vi "TestSimpleVISAconnection.vi"() -> ()   [LabVIEW 2015]
panel:
  out "read buffer":string
  in  "wr":bool
  in  "write buffer":string="*IDN?"
  in  "write":bool
  in  "VISA resource name":refnum<visa-resource-name>
  out "error out 2":errorcluster caption="error out" {"code" format="%.0x"}
  in  "stop":bool
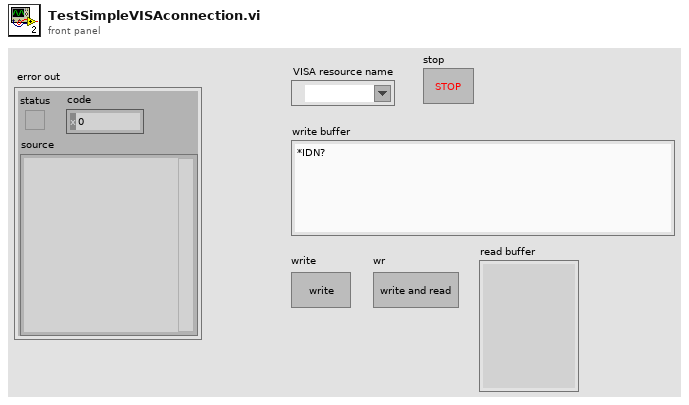
[diagram p1: front panel]
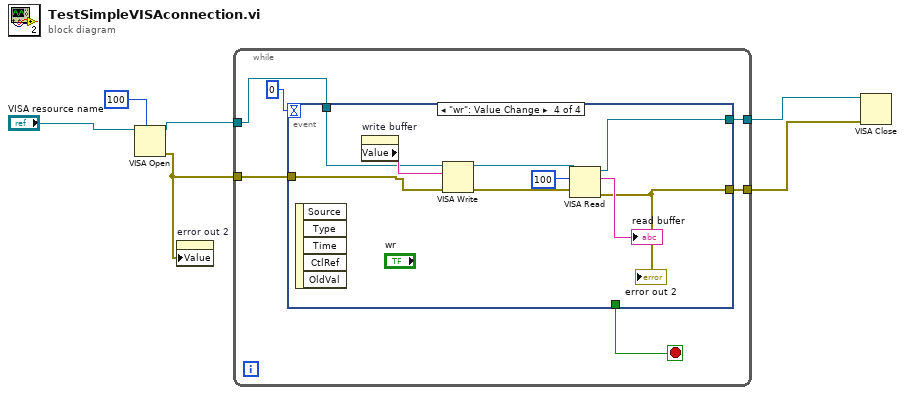
[diagram p0: block diagram]
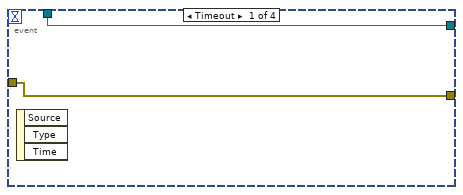
[diagram p2: hidden frame]
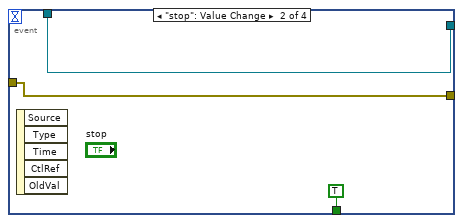
[diagram p3: hidden frame]
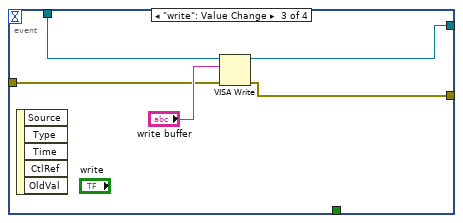
[diagram p4: hidden frame]
diagram:
  n1 = VISA Open(timeout (0)=u32 100 ("VISA Open timeout (0)"), VISA resource name="VISA resource name") -> (VISA resource name=w5:refnum<visa-resource-name>, error out=w1:errorcluster)  [unwired: 3 in]
  n2 = property on="error out 2" class="Clust (strict)"("Value"=w1) -> ()  [unwired: 2 in, 2 out]
  n3 = while {
    tunnel: w5 -> [w12]
    tunnel: [w9] -> w4
    tunnel: [w8] -> w2
    tunnel: w1 -> [w7]
    stop <- w10 stop-if-true
    n4 = event shown="[3] \"wr\": Value Change" {
      selector: _ -> [_ _ _ _]
      dyn-events: _ -> [_ _ _ _]
      timeout: 0 -> [_ _ _ _]
      tunnel: w12 -> [w14 w17 w22 w26]
      tunnel: [_ TRUE _ _] -> w10
      tunnel: [w14 w17 w21 w25] -> w9
      tunnel: [w13 w15 w19 w24] -> w8
      tunnel: w7 -> [w13 w15 w18 w23]
      event Timeout {
        n5 = event-data() -> ()  [unwired: 1 in, 3 out]
      }
      event "stop": Value Change {
        n6 = event-data() -> ()  [unwired: 1 in, 5 out]
      }
      event "write": Value Change {
        n7 = event-data() -> ()  [unwired: 1 in, 5 out]
        n8 = VISA Write(VISA resource name=w22, write buffer="write buffer", error in (no error)=w18) -> (VISA resource name out=w21:refnum<visa-resource-name>, error out=w19:errorcluster)  [unwired: 1 out]
      }
      event "wr": Value Change {
        n9 = event-data() -> ()  [unwired: 1 in, 5 out]
        n10 = property on="write buffer" class="Str"() -> ("Value"=w28:string)  [unwired: 2 in, 2 out]
        n11 = VISA Write(VISA resource name=w26, write buffer=w28, error in (no error)=w23) -> (VISA resource name out=w31:refnum<visa-resource-name>, error out=w29:errorcluster)  [unwired: 1 out]
        n12 = VISA Read(VISA resource name=w31, byte count=u32 100, error in (no error)=w29) -> (VISA resource name out=w25:refnum<visa-resource-name>, read buffer=→"read buffer":string, error out=w24:errorcluster)  [unwired: 1 out]
        "error out 2" <- w24
      }
    }
  }
  n13 = VISA Close(VISA resource name=w4, error in (no error)=w2) -> ()  [unwired: 1 out]
